vi "Multirecord Acquisition (FPGA)_20230126.vi"() -> ()   [LabVIEW 2021]
doc: "Use this VI as a template for the reconfigurable oscilloscope acquisition design. The block diagram is divided into three main loops.\n\nRegister Bus: This loop initializes the registers that are needed to support the configuration of the device. The FIFO bus, on the left, allows all the other design libraries to communicate with one another. This loop is very important to support the proper behavior of the instrument design library components.\n\nAcquisition: Acquires data from the I/O channels and writes the data into the record memory using the <B>Write</B> VI of the Multirecord Acquisition instrument design library. This VI also evaluates the various acquisition triggers and decides whether to acquire each data value in record memory. The host level VI (Fetch Record.vi) can read acquired records from the DRAM. The data is stored in 2 DRAM banks, each with 768 MB of storage.\n\nFetch: The recorded data is retrieved when the <B>Fetch Single Record</B> VI is run from the host VI. The <B>Write to Fetch DMA FIFO</B> VI writes data to the acq.fetch fifo 0 to transmit record data form the FPGA to the record fetch VIs on the host. This DMA FIFO must have a predefined name based on the instance parameter. By default, it is 0 (since the associated terminal on the <B>Create Resources DRAM Write Read</B> VI is unwired), so the connected FIFO is named acq.fetch fifo 0."
uses:
  <vilib>/Platform/TimedLoop/XDataNode/XDataNode.xnode
  <vilib>/Platform/TimedLoop/XDataNode/nitl_modes.ctl
  <vilib>/Platform/TimedLoop/XDataNode/XDNodeRunTimeDep.lvlib
  <vilib>/Platform/TimedLoop/XDataNode/wakeup.ctl
  <vilib>/Platform/TimedLoop/XDataNode/timing_clust.ctl
  <instrlib>/_niInstr/Multirecord Acquisition/Interface/v1/FPGA/niInstr Multirecord Acquisition v1 FPGA.lvclass
  <instrlib>/_niInstr/Multirecord Acquisition/Common/v1/FPGA/niInstr Multirecord Acquisition Common v1 FPGA.lvclass
  <vilib>/rvi/LocalResourceManager/LocalResourceManager.xnode
  <vilib>/rvi/eio/common/nirviEmuReportErrorAndStop.vi
  <vilib>/rvi/DataTransferAndStorage/Container/Common/niFpgaContainerGetUniqueNameForEmu.vi
  <vilib>/rvi/DataTransferAndStorage/Container/Common/niFpgaContainerSetEmuInfo.vi
  <vilib>/eio/EIONode/EIONode.xnode
  <instrlib>/_niInstr/FIFO Register Bus/v1/FPGA/niInstr FIFO Register Bus v1 FPGA.lvclass
  <instrlib>/_niInstr/Instruction Framework/v1/FPGA/Top Level Bus/Register Configuration/Register Configuration.lvclass
  <instrlib>/_niInstr/Channel/v1/FPGA/niInstr Channel v1 FPGA.lvlib
  <instrlib>/_niInstr/Basic Elements/v1/FPGA/niInstr Basic Elements v1 FPGA.lvlib
  <instrlib>/_niInstr/Multirecord Acquisition/Common/v1/FPGA/Private/Create Fetch DMA FIFO Resources U8x32.vi
  <instrlib>/HSAI-RIO/Config/Group A/v1/FPGA/Digital Correction/Digital Correction.lvclass
  <instrlib>/HSAI-RIO/Config/Group A/v1/FPGA/Config Registers/Config Registers.lvclass
  <instrlib>/_niInstr/Channel/v1/FPGA/Private/Select/Select FXP(+-,18,1,)xNspcx8ch.vi
  Trigger/Trigger FXP(+,-,18,1).vi
  <instrlib>/HSAI-RIO/Config/Group A/v1/FPGA/Digital Correction/FIR Filter (8 Ch).vi
  <instrlib>/_niInstr/Multirecord Acquisition/Interface/v1/FPGA/Private/Retrieve Record U16 Wrapper.vi
  <instrlib>/_niInstr/Multirecord Acquisition/Common/v1/FPGA/Private/Create Resources BRAM U384.vi
  <instrlib>/_niInstr/Multirecord Acquisition/Interface/v1/FPGA/Private/Write to Fetch DMA FIFO U16 Wrapper.vi
  <instrlib>/_niInstr/Multirecord Acquisition/Common/v1/FPGA/Private/Create Resources DRAM U384x2 U768 Write Read.vi
  Emulation/SubVIs/2 Element Generate Sine Cos Data FXP(+,-,14,1).vi
  <instrlib>/HSAI-RIO/Config/Group A/v1/FPGA/Digital Correction/Validate 8 Channel Data.vi
  <instrlib>/HSAI-RIO/Config/Group A/v1/FPGA/Digital Correction/Digital Correction (8 Ch).vi
  <instrlib>/_niInstr/Multirecord Acquisition/Common/v1/FPGA/Private/Create Resources DRAM U384.vi
  Data Type Conversion/SubVIs/Data Type Conversion FXP(+-,18,1) to I16x8ch.vi
  <instrlib>/_niInstr/Multirecord Acquisition/Common/v1/FPGA/Private/Create Resources BRAM U768.vi
  DSP/SubVIs/Integer decimationx8ch.vi
  <instrlib>/_niInstr/Multirecord Acquisition/Interface/v1/FPGA/Private/Write I16 Wrapper.vi
  <instrlib>/_niInstr/Channel/v1/FPGA/Private/Select and Interleave/Select And Interleave I16xNspcx8ch.vi
  C:/Program Files (x86)/National Instruments/LabVIEW 2021/instr.lib/_niInstr/Multirecord Acquisition/Interface/v1/FPGA/niInstr Multirecord Acquisition v1 FPGA.lvclass
  C:/Program Files (x86)/National Instruments/LabVIEW 2021/instr.lib/_niInstr/Multirecord Acquisition/Common/v1/FPGA/niInstr Multirecord Acquisition Common v1 FPGA.lvclass
  <vilib>/rvi/eio/common/nirviEmuTemplateMethod_errors.vi
  Data Type Conversion/SubVIs/Remove Overflow FXP(+-,18,1)x8ch.vi
  C:/Program Files (x86)/National Instruments/LabVIEW 2021/instr.lib/_niInstr/Instruction Framework/v1/FPGA/Interfaces/Instruction Producer/Instruction Producer.lvclass
  C:/Program Files (x86)/National Instruments/LabVIEW 2021/instr.lib/_niInstr/FIFO Register Bus/v1/FPGA/niInstr FIFO Register Bus v1 FPGA.lvclass
  FPGA Interface Typedefinitions/Trigger Combination Type.ctl
  FPGA Interface Typedefinitions/FPGA Interface Typedefinitions.lvlib
  <instrlib>/_niInstr/Data Trigger/v1/Shared/Public/Level Configuration FXP(+-,18,1).ctl
  <instrlib>/_niInstr/Data Trigger/v1/Shared/niInstr Data Trigger v1 Shared.lvlib
  <instrlib>/_niInstr/Data Trigger/v1/Shared/Public/Level Configuration Trigger When.ctl
panel:
  out "TrgdChan":u8
  in  "trig 7":cluster{"Hi":T1, "Lo":T1}
  in  "trig 6":cluster{"Hi":T1, "Lo":T1}
  in  "trig 5":cluster{"Hi":T1, "Lo":T1}
  in  "trig 4":cluster{"Hi":T1, "Lo":T1}
  in  "trig 3":cluster{"Hi":T1, "Lo":T1}
  in  "trig 2":cluster{"Hi":T1, "Lo":T1}
  in  "trig 1":cluster{"Hi":T1, "Lo":T1}
  in  "trig 0":cluster{"Hi":T1, "Lo":T1}
  in  "trigger.rearm delay":u16=2
  in  "start trigger":bool=TRUE
  in  "reset":bool
  in  "trigger.combination type":T3
  out "fifo reg bus data 0":u64
  out "fifo reg bus status 0":u32
  in  "fifo reg bus ctrl 0":u32
  out "overflow":bool
  in  "dsp.decimation factor":u16
  out "overload":bool
  in  "channel.enable mask":u16=65535 format="%.0b"
  in  "channel.number of channels":u8=8
  # "Register Bus Controls"
  # "FPGA"
  # "Acquisition Loop Controls"
  # "DSP"
  # "Trigger"
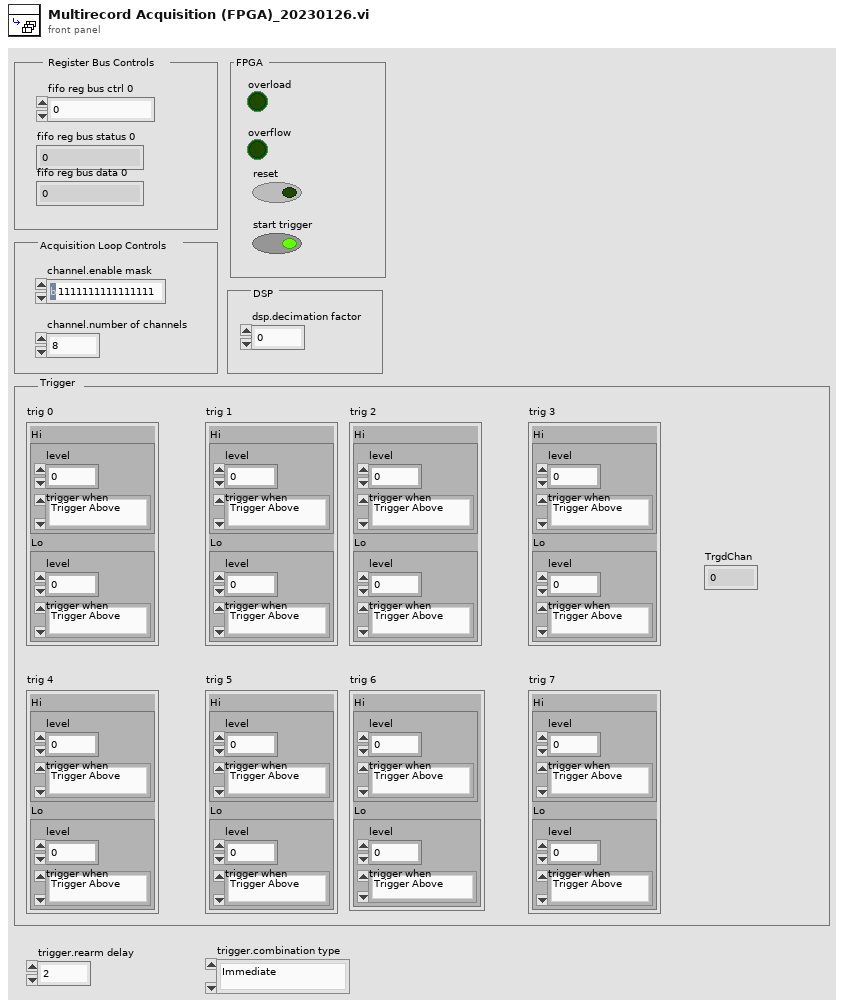
[diagram p1: front panel]
types:
  T1 = typedef "niInstr Data Trigger v1 Shared.lvlib/Level Configuration FXP(+-,18,1).ctl" = cluster{"level":fxp<+/-,18,1>, "trigger when":T2}
  T2 = typedef "niInstr Data Trigger v1 Shared.lvlib/Level Configuration Trigger When.ctl" = enum8{"Trigger Above", "Trigger Below"}
  T3 = typedef "FPGA Interface Typedefinitions.lvlib/Trigger Combination Type.ctl" = enum16{"Immediate", "A", "B", "OR", "AND", "A THEN B", "B THEN A", "High Resolution"}
  T4 = cluster{"memory 1":refnum<k21>, "memory 2":refnum<k21>}
  T5 = typedef "XDNodeRunTimeDep.lvlib/timing_clust.ctl" = cluster{"Expected End [f-1]":u64, "Actual End [f-1]":u64, "Finished Late? [f-1]":bool, "Expected End [i-1]":u64, "Actual End [i-1]":u64, "Finished Late? [i-1]":bool, "Expected Start [i]":u64, "Actual Start [i]":u64, "Expected Start [f]":u64, "Actual Start [f]":u64, "Source Name":string, "Structure Name":string, "Period":i64, "Deadline":i64, "Offset":i64, "Start":i64, "Priority":i32, "Timeout":i32, "Mode":T6, "Wakeup Reason":T7, "Error":errorcluster, "Source Type":string, "Secondary Source Type":string, "Global End Time":u64, "Global Start Time":u64, "Frame Duration":u64, "Iteration Duration":u64, "Assigned CPU":i32, "I/O Scan Engine Mode":u32}
  T6 = typedef "XDNodeRunTimeDep.lvlib/nitl_modes.ctl" = enum32{"No Change", "Process missed periods, maintain original phase", "Discard missed periods, maintain original phase", "Process missed periods, ignore original phase", "Discard missed periods, ignore original phase"}
  T7 = typedef "XDNodeRunTimeDep.lvlib/wakeup.ctl" = enum32{"Normal", "Aborted", "Asynchronous wakeup", "Timing source error", "Timed loop error", "Timeout"}
  T8 = cluster{"Channel 0":fxp<+/-,14,1>[], "Channel 1":fxp<+/-,14,1>[], "Channel 2":fxp<+/-,14,1>[], "Channel 3":fxp<+/-,14,1>[], "Channel 4":fxp<+/-,14,1>[], "Channel 5":fxp<+/-,14,1>[], "Channel 6":fxp<+/-,14,1>[], "Channel 7":fxp<+/-,14,1>[]}
  T9 = cluster{"Channel 0":fxp<+/-,18,1>[], "Channel 1":fxp<+/-,18,1>[], "Channel 2":fxp<+/-,18,1>[], "Channel 3":fxp<+/-,18,1>[], "Channel 4":fxp<+/-,18,1>[], "Channel 5":fxp<+/-,18,1>[], "Channel 6":fxp<+/-,18,1>[], "Channel 7":fxp<+/-,18,1>[]}
  T10 = cluster{"channel 0":fxp<+/-,18,1>[], "channel 1":fxp<+/-,18,1>[], "channel 2":fxp<+/-,18,1>[], "channel 3":fxp<+/-,18,1>[], "channel 4":fxp<+/-,18,1>[], "channel 5":fxp<+/-,18,1>[], "channel 6":fxp<+/-,18,1>[], "channel 7":fxp<+/-,18,1>[]}
  T11 = cluster{"channel 0":i16[], "channel 1":i16[], "channel 2":i16[], "channel 3":i16[], "channel 4":i16[], "channel 5":i16[], "channel 6":i16[], "channel 7":i16[]}
  T12 = typedef "niInstr Multirecord Acquisition v1 FPGA.lvclass/Timestamp.ctl" = cluster{"timestamp":u64, "valid":bool}
  T13 = typedef "niInstr Types v1 Shared.lvlib/Input Triggers.ctl" = cluster{"start":bool, "advance":bool, "reference":bool, "start trigger index":u16, "advance trigger index":u16, "reference trigger index":u16, "reference trigger correction cycle count":u32}
  T14 = typedef "niInstr Types v1 Shared.lvlib/Sample Format.ctl" = cluster{"bits per channel":u16, "samples per clock":u16, "channels":u8}
  T15 = typedef "niInstr Multirecord Acquisition v1 FPGA.lvclass/Events.ctl" = cluster{"ready for start":bool, "ready for advance":bool, "ready for reference":bool, "end of record":bool, "done":bool, "start trigger":bool, "advance trigger":bool, "reference trigger":bool, "start trigger index":u16, "advance trigger index":u16, "reference trigger index":u16}
  T16 = typedef "niInstr Multirecord Acquisition v1 FPGA.lvclass/Retrieve Data Info.ctl" = cluster{"read request size (bits)":u64, "valid data offset (bits)":u16, "valid data size (bits)":u16, "first sample of request":bool, "last sample of request":bool, "Token":T17}
  T17 = typedef "niInstr Types v1 Shared.lvlib/Token.ctl" = cluster{"identifier":u8, "value":u32}
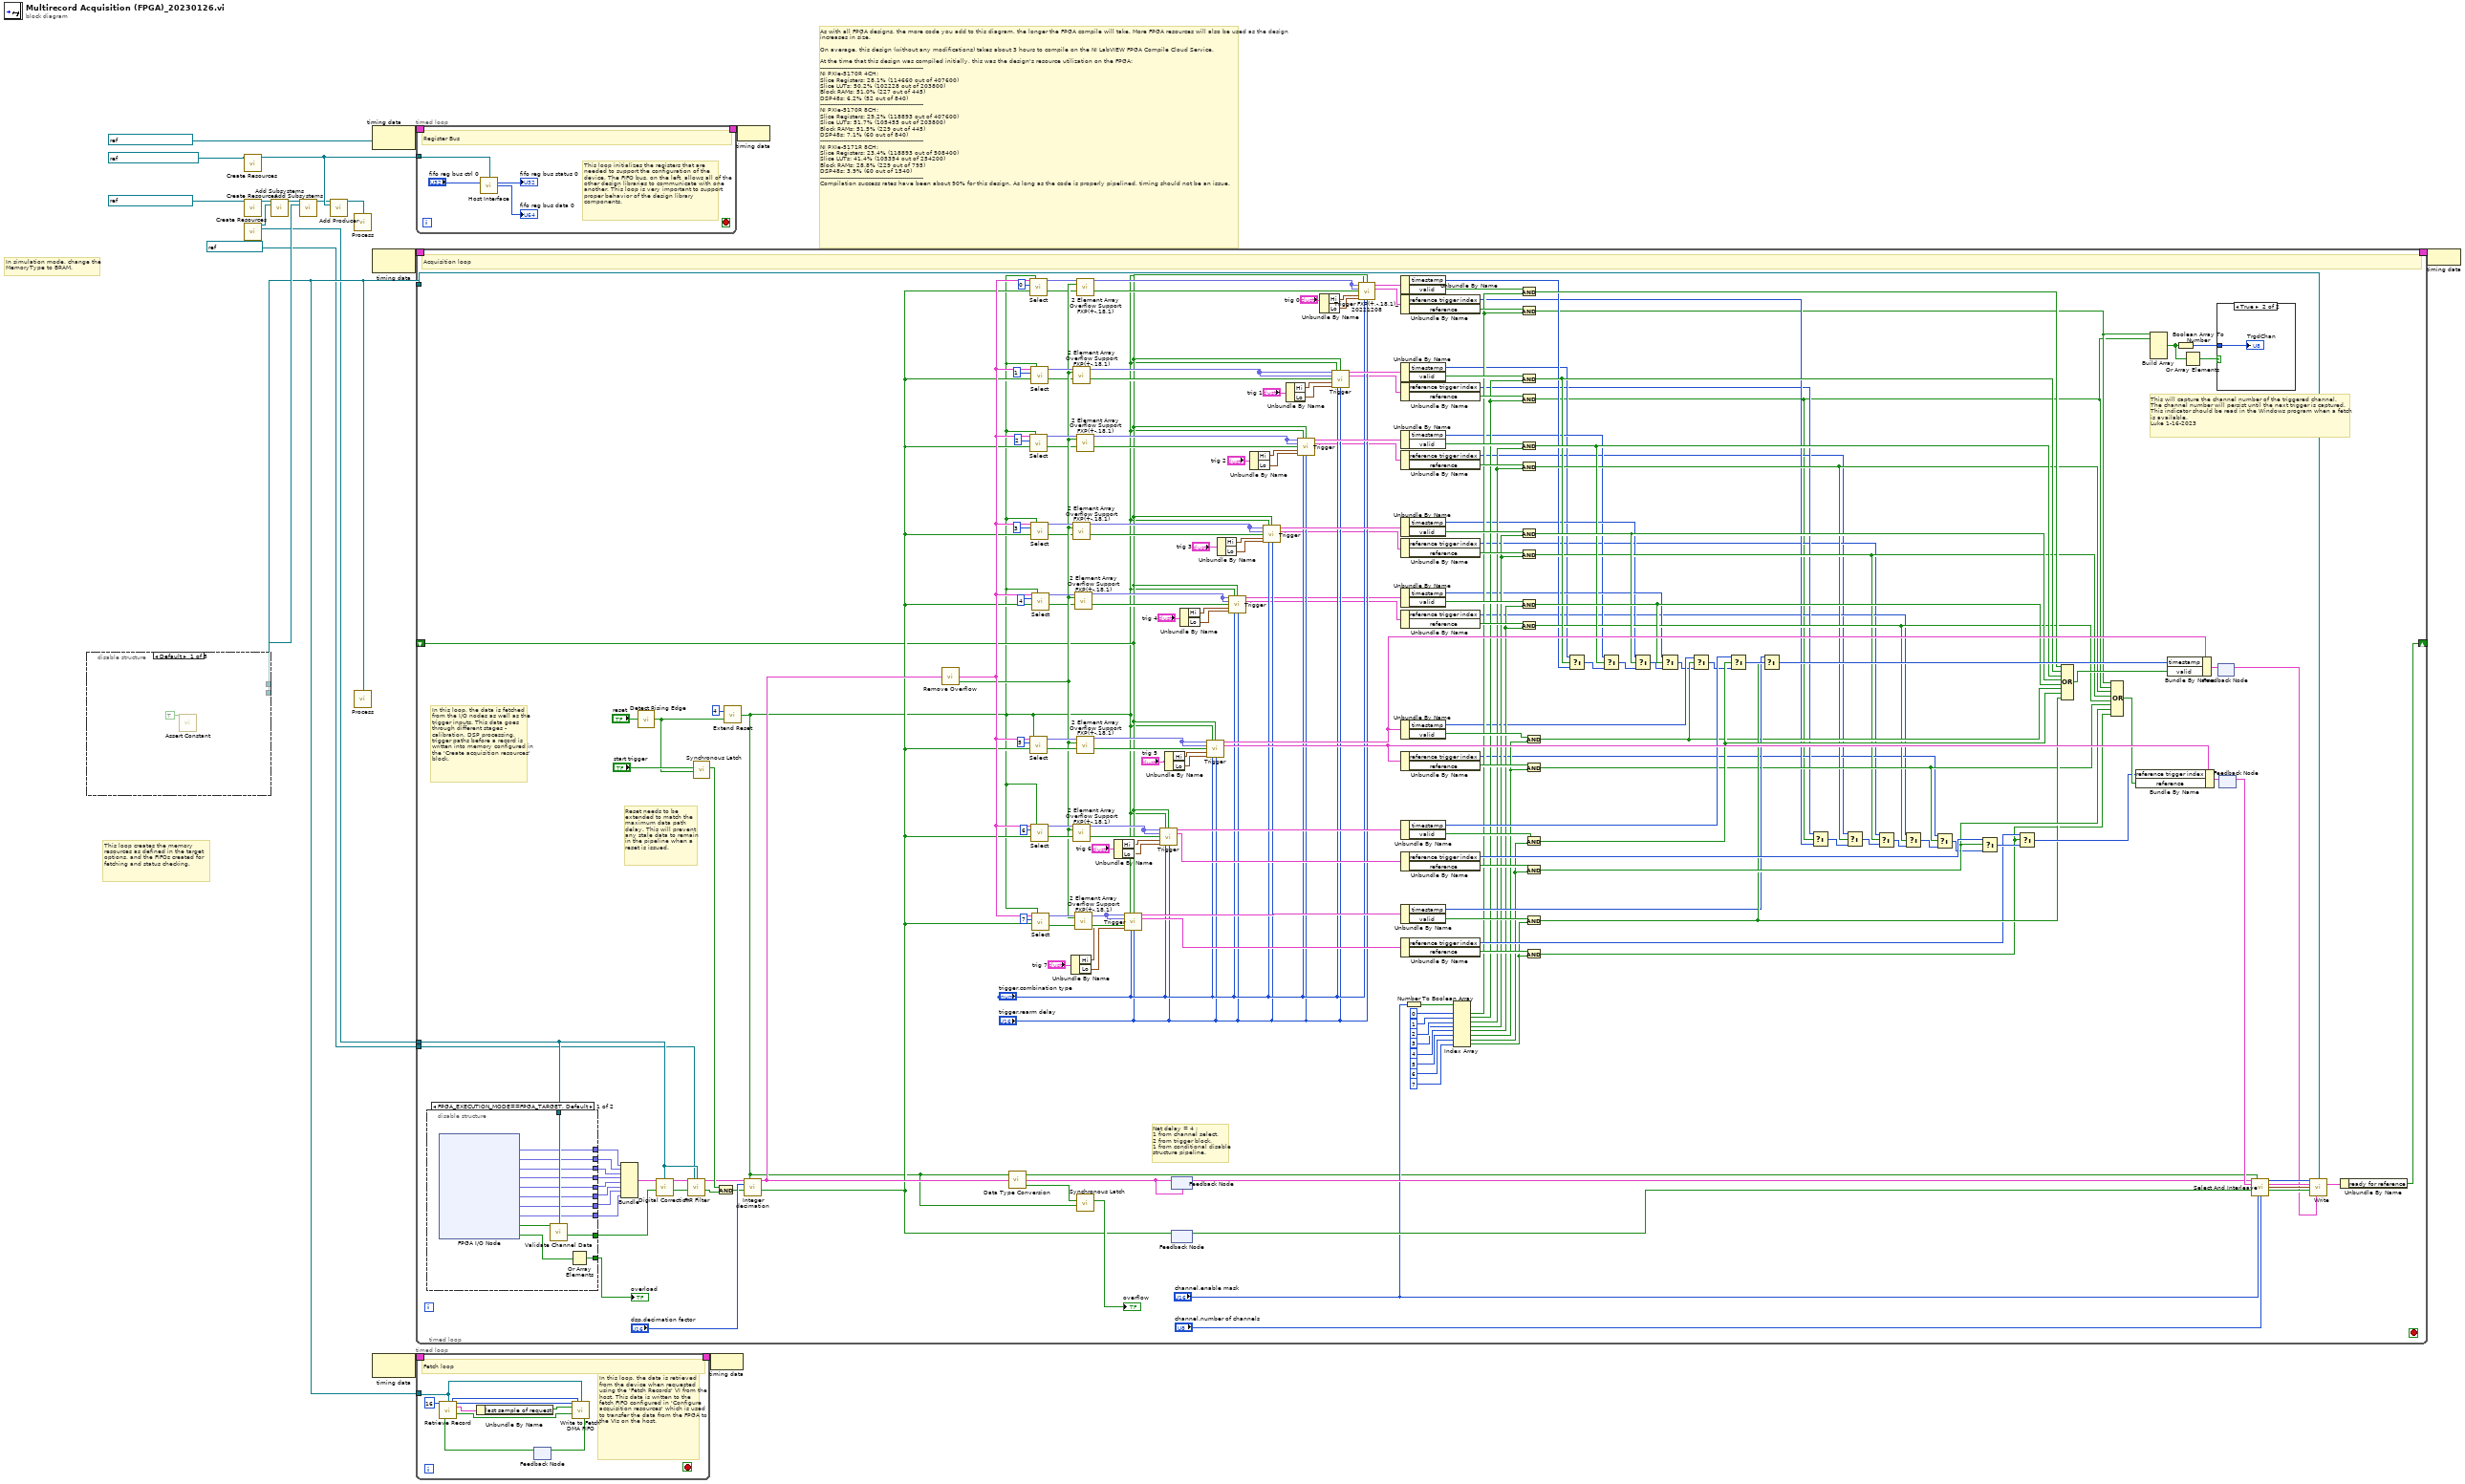
[diagram p0: block diagram]
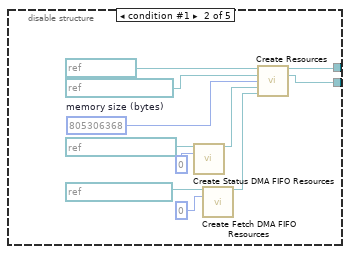
[diagram p2: hidden frame]
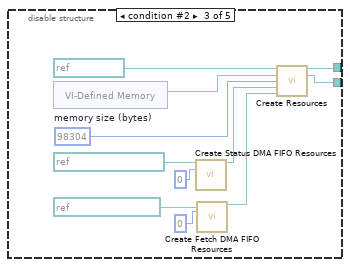
[diagram p3: hidden frame]
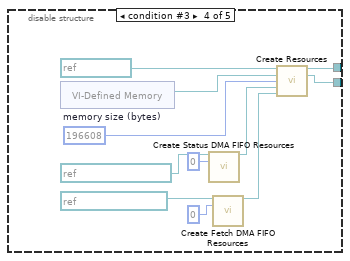
[diagram p4: hidden frame]
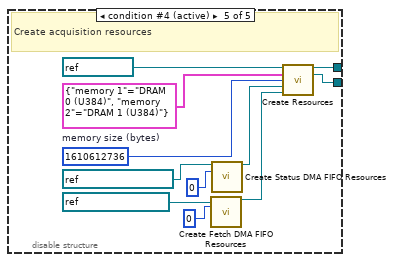
[diagram p5: hidden frame]
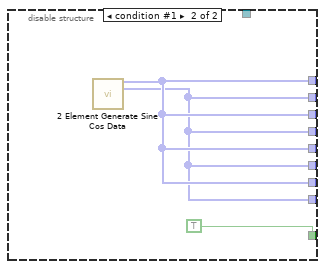
[diagram p7: hidden frame]
diagram:
  # "In simulation mode, change the MemoryType to BRAM."
  # "This loop creates the memory resources as defined in the target options, and the FIFOs created for fetching and status checking."
  # "As with all FPGA designs, the more code you add to this diagram, the longer the FPGA compile will take. More FPGA resources will also be used as the design increases in size.\n\nOn average, this design (without any modifications) takes about 3 hours to compile on the NI LabVIEW FPGA Compile Cloud Service. \n\nAt the time that this design was compiled initially, this was the design's resource utilization on the FPGA:\n------------------------------------------------------\nNI PXIe-5170R 4CH:\nSlice Registers: 28.1% (114660 out of 407600)\nSlice LUTs: 50.2% (102228 out of 203800)\nBlock RAMs: 51.0% (227 out of 445)\nDSP48s: 6.2% (52 out of 840)\n------------------------------------------------------\nNI PXIe-5170R 8CH:\nSlice Registers: 29.2% (118893 out of 407600)\nSlice LUTs: 51.7% (105455 out of 203800)\nBlock RAMs: 51.5% (229 out of 445)\nDSP48s: 7.1% (60 out of 840)\n------------------------------------------------------\nNI PXIe-5171R 8CH:\nSlice Registers: 23.4% (118893 out of 508400)\nSlice LUTs: 41.4% (105354 out of 254200)\nBlock RAMs: 28.8% (229 out of 795)\nDSP48s: 3.9% (60 out of 1540)\n------------------------------------------------------\nCompilation success rates have been about 90% for this design. As long as the code is properly pipelined, timing should not be an issue."
  n1 = disable-structure shown="Default" {
    disable-tunnel: [_ w29 w40 w51 w62] -> w4
    disable-tunnel: [_ w26 w36 w47 w59] -> w7
    frame condition #0 {
      n2 = call <instrlib>:"Assert Constant.vi"("constant terminal"=TRUE) -> ()  [unwired: 15 in]
    }
    frame condition #1 {
      w30 = u64 805306368  # memory size (bytes)
      n3 = call <instrlib>:"Create Status DMA FIFO Resources.vi"("status dma fifo in"=refnum<k21> "acq.status fifo 0" ("status dma fifo"), "fifo instance"=u8 0) -> ("status dma fifo out"=w21:refnum<class "niInstr Status FIFO v1 FPGA.lvclass">)  [unwired: 13 in]
      n4 = call-poly <instrlib>:"Create Fetch DMA FIFO Resources.vi"("fetch dma fifo in"=refnum<k21> "acq.fetch fifo 0", "fifo instance"=u8 0) -> ("fetch dma fifo out"=w27:refnum<class "niInstr Fetch FIFO v1 FPGA.lvclass">)  [unwired: 13 in]
      n5 = call-poly <instrlib>:"Create Resources.vi"("memory clock"=refnum<k21> "160MHz" ("process clock"), "memory"=refnum<k21> "DRAM 0 (U384)" ("dram"), "memory size (bytes)"=w30, "status dma fifo resources"=w21, "fetch dma fifo resources"=w27) -> ("acquisition resources"=w29:refnum<class "niInstr Multirecord Acquisition Common v1 FPGA.lvclass">, "acquisition subsystem"=w26:refnum<class "Address Space Collection.lvclass">)  [unwired: 9 in]
    }
    frame condition #2 {
      w41 = u64 98304  # memory size (bytes)
      n6 = xnode "VI-Defined Memory"() -> ("Memory Out"=w42:refnum<k21>)
      n7 = call <instrlib>:"Create Status DMA FIFO Resources.vi"("status dma fifo in"=refnum<k21> "acq.status fifo 0" ("status dma fifo"), "fifo instance"=u8 0) -> ("status dma fifo out"=w33:refnum<class "niInstr Status FIFO v1 FPGA.lvclass">)  [unwired: 13 in]
      n8 = call-poly <instrlib>:"Create Fetch DMA FIFO Resources.vi"("fetch dma fifo in"=refnum<k21> "acq.fetch fifo 0", "fifo instance"=u8 0) -> ("fetch dma fifo out"=w37:refnum<class "niInstr Fetch FIFO v1 FPGA.lvclass">)  [unwired: 13 in]
      n9 = call-poly <instrlib>:"Create Resources.vi"("memory clock"=refnum<k21> "160MHz" ("process clock"), "memory"=w42, "memory size (bytes)"=w41, "status dma fifo resources"=w33, "fetch dma fifo resources"=w37) -> ("acquisition resources"=w40:refnum<class "niInstr Multirecord Acquisition Common v1 FPGA.lvclass">, "acquisition subsystem"=w36:refnum<class "Address Space Collection.lvclass">)  [unwired: 9 in]
    }
    frame condition #3 {
      w52 = u64 196608  # memory size (bytes)
      n10 = xnode "VI-Defined Memory"() -> ("Memory Out"=w53:refnum<k21>)
      n11 = call <instrlib>:"Create Status DMA FIFO Resources.vi"("status dma fifo in"=refnum<k21> "acq.status fifo 0" ("status dma fifo"), "fifo instance"=u8 0) -> ("status dma fifo out"=w45:refnum<class "niInstr Status FIFO v1 FPGA.lvclass">)  [unwired: 13 in]
      n12 = call-poly <instrlib>:"Create Fetch DMA FIFO Resources.vi"("fetch dma fifo in"=refnum<k21> "acq.fetch fifo 0", "fifo instance"=u8 0) -> ("fetch dma fifo out"=w48:refnum<class "niInstr Fetch FIFO v1 FPGA.lvclass">)  [unwired: 13 in]
      n13 = call-poly <instrlib>:"Create Resources.vi"("memory clock"=refnum<k21> "160MHz" ("process clock"), "memory"=w53, "memory size (bytes)"=w52, "status dma fifo resources"=w45, "fetch dma fifo resources"=w48) -> ("acquisition resources"=w51:refnum<class "niInstr Multirecord Acquisition Common v1 FPGA.lvclass">, "acquisition subsystem"=w47:refnum<class "Address Space Collection.lvclass">)  [unwired: 9 in]
    }
    frame condition #4 (active) {
      w64 = u64 1610612736  # memory size (bytes)
      # "Create acquisition resources"
      n14 = call-poly <instrlib>:"Create Fetch DMA FIFO Resources.vi"("fetch dma fifo in"=refnum<k21> "acq.fetch fifo 0", "fifo instance"=u8 0) -> ("fetch dma fifo out"=w61:refnum<class "niInstr Fetch FIFO v1 FPGA.lvclass">)  [unwired: 13 in]
      n15 = call <instrlib>:"Create Status DMA FIFO Resources.vi"("status dma fifo in"=refnum<k21> "acq.status fifo 0" ("status dma fifo"), "fifo instance"=u8 0) -> ("status dma fifo out"=w56:refnum<class "niInstr Status FIFO v1 FPGA.lvclass">)  [unwired: 13 in]
      n16 = call-poly <instrlib>:"Create Resources.vi"("memory clock"=refnum<k21> "160MHz" ("process clock"), "memory"=T4 {"memory 1"="DRAM 0 (U384)", "memory 2"="DRAM 1 (U384)"}, "memory size (bytes)"=w64, "status dma fifo resources"=w56, "fetch dma fifo resources"=w61) -> ("acquisition resources"=w62:refnum<class "niInstr Multirecord Acquisition Common v1 FPGA.lvclass">, "acquisition subsystem"=w59:refnum<class "Address Space Collection.lvclass">)  [unwired: 9 in]
    }
  }
  n17 = call <instrlib>:"Create Resources.vi"("instruction fifo"=refnum<k21> "reg.host instruction fifo 0" ("FIFO")) -> ("fifo register bus"=w6:refnum<class "niInstr FIFO Register Bus v1 FPGA.lvclass">)  [unwired: 14 in]
  n18 = call <instrlib>:"Create Resources.vi"("register clock"=refnum<k21> "40 MHz Onboard Clock" ("Source Name")) -> ("register configuration"=w10:refnum<class "Register Configuration.lvclass">)  [unwired: 14 in]
  n19 = call <instrlib>:"Create Resources.vi"() -> ("config subsystems"=w8:refnum<class "Address Space Collection.lvclass">, "digital correction resources"=w1:refnum<class "Digital Correction.lvclass">)  [unwired: 14 in]
  n20 = call-dynamic "Add Subsystems.vi"("register configuration in"=w10, "subsystems"=w8) -> ("register configuration out"=w9:refnum<class "Register Configuration.lvclass">)  [unwired: 13 in]
  n21 = call-dynamic "Add Subsystems.vi"("register configuration in"=w9, "subsystems"=w7) -> ("register configuration out"=w3:refnum<class "Register Configuration.lvclass">)  [unwired: 13 in]
  n22 = call-dynamic "Add Producer.vi"("register configuration in"=w3, "instruction producer"=w6) -> ("register configuration out"=w5:refnum<class "Register Configuration.lvclass">)  [unwired: 13 in]
  n23 = call-dynamic "Process.vi"("register configuration"=w5) -> ()  [unwired: 15 in]
  n24 = call-dynamic "Process.vi"("acquisition resources"=w4) -> ()  [unwired: 15 in]
  n25 = node-c288(refnum<k21> "40 MHz Onboard Clock" ("Source Name")) -> (w19:T5)
  n26 = node-c288() -> (w17:T5)  [unwired: 1 in]
  n27 = node-c288() -> (w15:T5)  [unwired: 1 in]
  n28 = timed-loop {
    timing: w19 -> [_]
    timing-out: [_] -> w18
    tunnel: w6 -> [w68]
    stop <- _ stop-if-true
    # "This loop initializes the registers that are needed to support the configuration of the device. The FIFO bus, on the left, allows all of the other design libraries to communicate with one another. This loop is very important to support proper behavior of the design library components."
    # "Register Bus"
    n29 = call <instrlib>:"Host Interface.vi"("fifo register bus"=w68, "fifo reg bus ctrl 0"="fifo reg bus ctrl 0") -> ("fifo reg bus status 0"=→"fifo reg bus status 0":u32, "fifo reg bus data 0"=→"fifo reg bus data 0":u64)  [unwired: 12 in]
  }
  n30 = timed-loop {
    timing: w17 -> [_]
    timing-out: [_] -> w16
    tunnel: w4 -> [w275]
    tunnel: w1 -> [w258]
    shift-right: [w267] -> _
    shift-left: _ -> [w170]
    tunnel: refnum<k21> "Data Clock x2" -> [w255]
    stop <- _ stop-if-true
    # "This will capture the channel number of the triggered channel.\nThe channel number will persist until the next trigger is captured.\nThis indicator should be read in the Windows program when a fetch\nis available.\nLuke 1-16-2023"
    # "Net delay = 4 :\n1 from channel select.\n2 from trigger block.\n1 from conditional disable structure pipeline."
    # "Reset needs to be extended to match the maximum data path delay. This will prevent any stale data to remain in the pipeline when a reset is issued."
    # "In this loop, the data is fetched from the I/O nodes as well as the trigger inputs. This data goes through different stages - calibration, DSP processing, trigger paths before a record is written into memory configured in the 'Create acquisition resources' block."
    # "Acquisition loop"
    n31 = disable-structure shown="FPGA_EXECUTION_MODE==FPGA_TARGET, Default" {
      disable-tunnel: [w288 w293] -> w254
      disable-tunnel: [w287 w292] -> w253
      disable-tunnel: [w286 w293] -> w252
      disable-tunnel: [w285 w292] -> w251
      disable-tunnel: [w284 w293] -> w250
      disable-tunnel: [w283 w292] -> w249
      disable-tunnel: [w282 w293] -> w247
      disable-tunnel: [w281 w292] -> w248
      disable-tunnel: [w278 TRUE ("ADC Data Valid")] -> w245
      disable-tunnel: w258 -> [w289 _]
      disable-tunnel: [w279 _] -> w274
      frame condition #0 (active) {
        # "I/O Nodes"
        n32 = xnode "FPGA I/O Node"() -> ("Channel 0"=w288:fxp<+/-,14,1>[], "Channel 1"=w287:fxp<+/-,14,1>[], "Channel 2"=w286:fxp<+/-,14,1>[], "Channel 3"=w285:fxp<+/-,14,1>[], "Channel 4"=w284:fxp<+/-,14,1>[], "Channel 5"=w283:fxp<+/-,14,1>[], "Channel 6"=w282:fxp<+/-,14,1>[], "Channel 7"=w281:fxp<+/-,14,1>[], "Channel Data Valid"=w290:bool[], "Channel Overload"=w280:bool[])  [unwired: 10 in, 10 out]
        n33 = call-poly <instrlib>:"Validate Channel Data.vi"("channel data valid"=w290, "digital correction resources"=w289) -> ("expected data valid"=w278:bool)  [unwired: 13 in]
        n34 = Or Array Elements(Boolean array=w280) -> (logical OR=w279:bool)
      }
      frame condition #1 {
        n35 = call-poly "2 Element Generate Sine Cos Data.vi"() -> ("sine data"=w293:fxp<+/-,14,1>[], "cosine data"=w292:fxp<+/-,14,1>[])  [unwired: 14 in]
      }
    }
    "overload" <- w274
    n36 = Bundle("Channel 0"=w254, "Channel 1"=w253, "Channel 2"=w252, "Channel 3"=w251, "Channel 4"=w250, "Channel 5"=w249, "Channel 6"=w247, "Channel 7"=w248) -> (w246:T8)  [unwired: 1 in]
    n37 = call <instrlib>:"Detect Rising Edge.vi"("signal"="reset") -> ("edge detected"=w257:bool)  [unwired: 14 in]
    n38 = call-poly <instrlib>:"Digital Correction.vi"("channel data in"=w246, "digital correction resources"=w258, "input valid"=w245) -> ("corrected channel data out"=w238:T9, "output valid"=w237:bool)  [unwired: 11 in]
    n39 = call-poly <instrlib>:"FIR Filter.vi"("data in"=w238, "data clock x2"=w255, "digital correction resources"=w258, "input valid"=w237) -> ("data out"=w235:T9, "output valid"=w236:bool)  [unwired: 9 in, 1 out]
    n40 = call <instrlib>:"Synchronous Latch.vi"("clear"=w257, "set"="start trigger") -> ("out"=w263:bool)  [unwired: 9 in]
    n41 = And(x=w263, y=w236) -> (x .and. y?=w239:bool)
    n42 = call "Extend Reset.vi"("reset in"=w257, "number of cycles"=u8 4) -> ("reset out"=w76:bool)
    n43 = call-poly "Integer decimation.vi"("data in"=w235, "reset"=w76, "decimation factor"="dsp.decimation factor", "input valid"=w239) -> ("data out"=w242:T10, "output valid"=w186:bool)  [unwired: 9 in, 1 out]
    n44 = call-poly "Remove Overflow.vi"("data in"=w242) -> ("overflow"=w180:bool, "data out"=w192:T10)  [unwired: 3 in]
    n45 = call-poly "Data Type Conversion.vi"("data in"=w242) -> ("overflow"=w244:bool, "data out"=w241:T11)  [unwired: 3 in]
    n46 = call-poly <instrlib>:"Select.vi"("data in"=w192, "reset"=w76, "channel index"=u8 0 ("trigger.channel A"), "input valid"=w186) -> ("channel out"=w191:fxp<+/-,18,1>[], "output valid"=w175:bool)  [unwired: 10 in]
    n47 = call-poly <instrlib>:"Select.vi"("data in"=w192, "reset"=w76, "channel index"=u8 2 ("trigger.channel A"), "input valid"=w186) -> ("channel out"=w189:fxp<+/-,18,1>[], "output valid"=w177:bool)  [unwired: 10 in]
    n48 = call-poly <instrlib>:"Select.vi"("data in"=w192, "reset"=w76, "channel index"=u8 5 ("trigger.channel A"), "input valid"=w186) -> ("channel out"=w265:fxp<+/-,18,1>[], "output valid"=w234:bool)  [unwired: 10 in]
    n49 = call-poly <instrlib>:"Select.vi"("data in"=w192, "reset"=w76, "channel index"=u8 1, "input valid"=w186) -> ("channel out"=w190:fxp<+/-,18,1>[], "output valid"=w176:bool)  [unwired: 10 in]
    n50 = call-poly <instrlib>:"Select.vi"("data in"=w192, "reset"=w76, "channel index"=u8 3, "input valid"=w186) -> ("channel out"=w188:fxp<+/-,18,1>[], "output valid"=w178:bool)  [unwired: 10 in]
    n51 = call-poly <instrlib>:"Select.vi"("data in"=w192, "reset"=w76, "channel index"=u8 6, "input valid"=w186) -> ("channel out"=w231:fxp<+/-,18,1>[], "output valid"=w229:bool)  [unwired: 10 in]
    n52 = call-poly <instrlib>:"Select.vi"("data in"=w192, "reset"=w76, "channel index"=u8 4, "input valid"=w186) -> ("channel out"=w187:fxp<+/-,18,1>[], "output valid"=w179:bool)  [unwired: 10 in]
    n53 = call-poly <instrlib>:"Select.vi"("data in"=w192, "reset"=w76, "channel index"=u8 7, "input valid"=w186) -> ("channel out"=w210:fxp<+/-,18,1>[], "output valid"=w208:bool)  [unwired: 10 in]
    n54 = Unbundle By Name("trig 7") -> ("Hi"=w78:T1, "Lo"=w77:T1)
    n55 = call "2 Element Array Overflow Support FXP(+-,18,1).vi"("data in"=w190, "overflow"=w180) -> ("data out"=w184:fxp<+/-,18,1>[])  [unwired: 13 in]
    n56 = call "2 Element Array Overflow Support FXP(+-,18,1).vi"("data in"=w188, "overflow"=w180) -> ("data out"=w182:fxp<+/-,18,1>[])  [unwired: 13 in]
    n57 = call "2 Element Array Overflow Support FXP(+-,18,1).vi"("data in"=w231, "overflow"=w180) -> ("data out"=w230:fxp<+/-,18,1>[])  [unwired: 13 in]
    n58 = call "2 Element Array Overflow Support FXP(+-,18,1).vi"("data in"=w187, "overflow"=w180) -> ("data out"=w181:fxp<+/-,18,1>[])  [unwired: 13 in]
    n59 = call "2 Element Array Overflow Support FXP(+-,18,1).vi"("data in"=w210, "overflow"=w180) -> ("data out"=w209:fxp<+/-,18,1>[])  [unwired: 13 in]
    n60 = call "2 Element Array Overflow Support FXP(+-,18,1).vi"("data in"=w191, "overflow"=w180) -> ("data out"=w185:fxp<+/-,18,1>[])  [unwired: 13 in]
    n61 = call "2 Element Array Overflow Support FXP(+-,18,1).vi"("data in"=w189, "overflow"=w180) -> ("data out"=w183:fxp<+/-,18,1>[])  [unwired: 13 in]
    n62 = call "2 Element Array Overflow Support FXP(+-,18,1).vi"("data in"=w265, "overflow"=w180) -> ("data out"=w233:fxp<+/-,18,1>[])  [unwired: 13 in]
    n63 = call <instrlib>:"Synchronous Latch.vi"("clear"=w76, "set"=w244) -> ("out"=→"overflow":bool)  [unwired: 9 in]
    n64 = Unbundle By Name("trig 6") -> ("Hi"=w81:T1, "Lo"=w80:T1)
    n65 = call-poly "Trigger.vi"("data A"=w209, "reset"=w76, "trigger.ready for reference"=w170, "data B"=w209, "input valid"=w208, "trigger.level Hi"=w78, "trigger.level Lo"=w77, "trigger.combination type"="trigger.combination type", "rearm delay"="trigger.rearm delay") -> ("timestamps"=w207:T12, "trigger.out"=w206:T13)  [unwired: 4 in, 1 out]
    n66 = call-poly "Trigger.vi"("data A"=w230, "reset"=w76, "trigger.ready for reference"=w170, "data B"=w230, "input valid"=w229, "trigger.level Hi"=w81, "trigger.level Lo"=w80, "trigger.combination type"="trigger.combination type", "rearm delay"="trigger.rearm delay") -> ("timestamps"=w224:T12, "trigger.out"=w223:T13)  [unwired: 4 in, 1 out]
    n67 = Unbundle By Name("trig 5") -> ("Hi"=w84:T1, "Lo"=w83:T1)
    n68 = feedback #1(w241) -> (w243:T11)
    n69 = feedback-in #1(w241) -> ()
    n70 = feedback #2() -> (w240:bool)  [unwired: 1 in]
    n71 = feedback-in #2(w186) -> ()
    n72 = Unbundle By Name("trig 4") -> ("Hi"=w87:T1, "Lo"=w86:T1)
    n73 = call-poly "Trigger.vi"("data A"=w233, "reset"=w76, "trigger.ready for reference"=w170, "data B"=w233, "input valid"=w234, "trigger.level Hi"=w84, "trigger.level Lo"=w83, "trigger.combination type"="trigger.combination type", "rearm delay"="trigger.rearm delay") -> ("timestamps"=w228:T12, "trigger.out"=w226:T13)  [unwired: 4 in, 1 out]
    n74 = Unbundle By Name("trig 3") -> ("Hi"=w90:T1, "Lo"=w89:T1)
    n75 = call-poly "Trigger.vi"("data A"=w181, "reset"=w76, "trigger.ready for reference"=w170, "data B"=w181, "input valid"=w179, "trigger.level Hi"=w87, "trigger.level Lo"=w86, "trigger.combination type"="trigger.combination type", "rearm delay"="trigger.rearm delay") -> ("timestamps"=w163:T12, "trigger.out"=w162:T13)  [unwired: 4 in, 1 out]
    n76 = Unbundle By Name("trig 2") -> ("Hi"=w93:T1, "Lo"=w92:T1)
    n77 = call-poly "Trigger.vi"("data A"=w182, "reset"=w76, "trigger.ready for reference"=w170, "data B"=w182, "input valid"=w178, "trigger.level Hi"=w90, "trigger.level Lo"=w89, "trigger.combination type"="trigger.combination type", "rearm delay"="trigger.rearm delay") -> ("timestamps"=w171:T12, "trigger.out"=w164:T13)  [unwired: 4 in, 1 out]
    n78 = Unbundle By Name("trig 1") -> ("Hi"=w96:T1, "Lo"=w95:T1)
    n79 = call-poly "Trigger.vi"("data A"=w183, "reset"=w76, "trigger.ready for reference"=w170, "data B"=w183, "input valid"=w177, "trigger.level Hi"=w93, "trigger.level Lo"=w92, "trigger.combination type"="trigger.combination type", "rearm delay"="trigger.rearm delay") -> ("timestamps"=w172:T12, "trigger.out"=w165:T13)  [unwired: 4 in, 1 out]
    n80 = Unbundle By Name("trig 0") -> ("Hi"=w99:T1, "Lo"=w98:T1)
    n81 = call-poly "Trigger.vi"("data A"=w184, "reset"=w76, "trigger.ready for reference"=w170, "data B"=w184, "input valid"=w176, "trigger.level Hi"=w96, "trigger.level Lo"=w95, "trigger.combination type"="trigger.combination type", "rearm delay"="trigger.rearm delay") -> ("timestamps"=w173:T12, "trigger.out"=w166:T13)  [unwired: 4 in, 1 out]
    n82 = call "Trigger FXP(+,-,18,1)_20221208.vi"("data A"=w185, "reset"=w76, "trigger.ready for reference"=w170, "data B"=w185, "input valid"=w175, "trigger.level Hi"=w99, "trigger.level Lo"=w98, "trigger.combination type"="trigger.combination type", "rearm delay"="trigger.rearm delay") -> ("timestamps"=w174:T12, "trigger.out"=w167:T13)  [unwired: 4 in, 1 out]
    n83 = Unbundle By Name(w174) -> ("timestamp"=w127:u64, "valid"=w156:bool)
    n84 = Unbundle By Name(w167) -> ("reference trigger index"=w116:u16, "reference"=w155:bool)
    n85 = Unbundle By Name(w173) -> ("timestamp"=w117:u64, "valid"=w154:bool)
    n86 = Unbundle By Name(w166) -> ("reference trigger index"=w115:u16, "reference"=w153:bool)
    n87 = Unbundle By Name(w172) -> ("timestamp"=w118:u64, "valid"=w152:bool)
    n88 = Unbundle By Name(w165) -> ("reference trigger index"=w106:u16, "reference"=w151:bool)
    n89 = Unbundle By Name(w171) -> ("timestamp"=w119:u64, "valid"=w150:bool)
    n90 = Unbundle By Name(w164) -> ("reference trigger index"=w107:u16, "reference"=w149:bool)
    n91 = Unbundle By Name(w163) -> ("timestamp"=w120:u64, "valid"=w148:bool)
    n92 = Unbundle By Name(w162) -> ("reference trigger index"=w108:u16, "reference"=w147:bool)
    n93 = Unbundle By Name(w228) -> ("timestamp"=w126:u64, "valid"=w216:bool)
    n94 = Unbundle By Name(w226) -> ("reference trigger index"=w110:u16, "reference"=w214:bool)
    n95 = Unbundle By Name(w224) -> ("timestamp"=w222:u64, "valid"=w215:bool)
    n96 = Unbundle By Name(w223) -> ("reference trigger index"=w221:u16, "reference"=w213:bool)
    n97 = Unbundle By Name(w207) -> ("timestamp"=w194:u64, "valid"=w204:bool)
    n98 = Unbundle By Name(w206) -> ("reference trigger index"=w193:u16, "reference"=w205:bool)
    n99 = Number To Boolean Array(number="channel.enable mask") -> (Boolean array=w219:bool[])
    n100 = Index Array(array=w219, index #1=0 ("index"), index #2=1 ("index"), index #3=2 ("index"), index #4=3 ("index"), index #5=4 ("index"), index #6=5 ("index"), index #7=6 ("index"), index #8=7 ("index")) -> (element #1=w146:bool, element #2=w145:bool, element #3=w144:bool, element #4=w143:bool, element #5=w142:bool, element #6=w141:bool, element #7=w140:bool, element #8=w139:bool)
    n101 = And(x=w156, y=w146) -> (x .and. y?=w137:bool)
    n102 = And(x=w155, y=w146) -> (x .and. y?=w75:bool)
    n103 = And(x=w154, y=w145) -> (x .and. y?=w132:bool)
    n104 = And(x=w153, y=w145) -> (x .and. y?=w74:bool)
    n105 = And(x=w152, y=w144) -> (x .and. y?=w133:bool)
    n106 = And(x=w151, y=w144) -> (x .and. y?=w128:bool)
    n107 = And(x=w150, y=w143) -> (x .and. y?=w134:bool)
    n108 = And(x=w149, y=w143) -> (x .and. y?=w129:bool)
    n109 = And(x=w148, y=w142) -> (x .and. y?=w135:bool)
    n110 = And(x=w147, y=w142) -> (x .and. y?=w130:bool)
    n111 = And(x=w216, y=w141) -> (x .and. y?=w136:bool)
    n112 = And(x=w214, y=w141) -> (x .and. y?=w131:bool)
    n113 = And(x=w215, y=w140) -> (x .and. y?=w203:bool)
    n114 = And(x=w213, y=w140) -> (x .and. y?=w201:bool)
    n115 = And(x=w204, y=w139) -> (x .and. y?=w195:bool)
    n116 = And(x=w205, y=w139) -> (x .and. y?=w138:bool)
    n117 = Select(t=w117, s=w132, f=w127) -> (s? t:f=w121:u64)
    n118 = Select(t=w118, s=w133, f=w121) -> (s? t:f=w122:u64)
    n119 = Select(t=w119, s=w134, f=w122) -> (s? t:f=w123:u64)
    n120 = Select(t=w120, s=w135, f=w123) -> (s? t:f=w124:u64)
    n121 = Select(t=w126, s=w136, f=w124) -> (s? t:f=w125:u64)
    n122 = Select(t=w222, s=w203, f=w125) -> (s? t:f=w199:u64)
    n123 = Select(t=w194, s=w195, f=w199) -> (s? t:f=w198:u64)
    n124 = Select(t=w115, s=w74, f=w116) -> (s? t:f=w114:u16)
    n125 = Select(t=w106, s=w128, f=w114) -> (s? t:f=w113:u16)
    n126 = Select(t=w107, s=w129, f=w113) -> (s? t:f=w112:u16)
    n127 = Select(t=w108, s=w130, f=w112) -> (s? t:f=w111:u16)
    n128 = Select(t=w110, s=w131, f=w111) -> (s? t:f=w109:u16)
    n129 = Select(t=w221, s=w201, f=w109) -> (s? t:f=w197:u16)
    n130 = Select(t=w193, s=w138, f=w197) -> (s? t:f=w196:u16)
    n131 = Compound Arithmetic op=OR(w137, w132, w133, w134, w135, w136, w203, w195) -> (w202:bool)
    n132 = Compound Arithmetic op=OR(w75, w74, w128, w129, w130, w131, w201, w138) -> (w200:bool)
    n133 = Bundle By Name(cluster=w226, "reference trigger index"=w196, "reference"=w200) -> (w225:T13)
    n134 = Build Array(w75, w74) -> (w72:bool[])  [unwired: 4 in]
    n135 = Bundle By Name(cluster=w228, "timestamp"=w198, "valid"=w202) -> (w227:T12)
    n136 = Boolean Array To Number(Boolean array=w72) -> (number=w73:u8)
    n137 = Or Array Elements(Boolean array=w72) -> (logical OR=w71:bool)
    n138 = case shown="True" w71 {
      tunnel: w73 -> [_ w277]
      frame False {
      }
      frame True {
        "TrgdChan" <- w277
      }
    }
    n139 = feedback #3() -> (w261:T12)  [unwired: 1 in]
    n140 = feedback-in #3(w227) -> ()
    n141 = feedback #4() -> (w262:T13)  [unwired: 1 in]
    n142 = feedback-in #4(w225) -> ()
    n143 = call-poly <instrlib>:"Select And Interleave.vi"("data in"=w243, "reset"=w76, "triggers in"=w262, "input valid"=w240, "channel enable mask"="channel.enable mask", "number of channels to interleave"="channel.number of channels") -> ("interleaved data out"=w273:i16[], "triggers out"=w272:T13, "sample format out"=w271:T14, "output valid"=w270:bool)  [unwired: 5 in, 1 out]
    n144 = call-poly <instrlib>:"Write.vi"("data"=w273, "acquisition resources"=w275, "triggers"=w272, "sample format"=w271, "data valid"=w270, "timestamp"=w261) -> ("events"=w268:T15)  [unwired: 7 in, 2 out]
    n145 = Unbundle By Name(w268) -> ("ready for reference"=w267:bool)
  }
  n146 = timed-loop {
    timing: w15 -> [_]
    timing-out: [_] -> w14
    tunnel: w4 -> [w304]
    stop <- _ stop-if-true
    # "In this loop, the data is retrieved from the device when requested using the 'Fetch Records' VI from the host. This data is written to the fetch FIFO configured in 'Configure acquisition resources' which is used to transfer the data from the FPGA to the VIs on the host."
    # "Fetch loop"
    n147 = feedback #5() -> (w302:bool)  [unwired: 1 in]
    n148 = call-poly <instrlib>:"Retrieve Record.vi"("output array size"=u16 16, "acquisition resources"=w304, "ready for output"=w302) -> ("channels"=w297:u8, "data"=w300:u16[], "retrieve data info"=w299:T16, "output valid"=w301:bool)  [unwired: 9 in]
    n149 = Unbundle By Name(w299) -> ("last sample of request"=w298:bool)
    n150 = call-poly <instrlib>:"Write to Fetch DMA FIFO.vi"("data"=w300, "channels"=w297, "acquisition resources"=w304, "last sample of request"=w298, "input valid"=w301) -> ("ready for input"=w303:bool)  [unwired: 10 in]
    n151 = feedback-in #5(w303) -> ()
  }
  n152 = node-c288(w14) -> ()
  n153 = node-c288(w18) -> ()
  n154 = node-c288(w16) -> ()
